vi "Projectile.vi"() -> ()   [LabVIEW 2014]
uses:
  <vilib>/imath/engines/lvmath2/RunTimeEngine/Managers/WorkSpace/UID Generator.vi
  <vilib>/imath/engines/lvmath2/RunTimeEngine/RunTimeType/NIMS_RunTimeType_From StrictType (excl LVString).vi
  <instcachedir>/0/NIMS_RunTimeType_From StrictType (excl LVString)_15A5391EEA9C4AACB9955AC755B83D29.lvgen/NIMS_RunTimeType_From StrictType (excl LVString)_15A5391EEA9C4AACB9955AC755B83D29_000.vi
  <vilib>/imath/engines/lvmath2/RunTimeEngine/LocalVariableDefStatement/MC_LocalVariableDefStatement_Display.vi
  <vilib>/imath/engines/lvmath2/RunTimeEngine/Managers/SymbolTable/Clear UID.vi
  <vilib>/imath/engines/lvmath2/RunTimeEngine/NodeEndStatement/NIMS_NodeEndStatement_Output.vi
  <instcachedir>/0/NIMS_NodeEndStatement_Output_53EC0D466D134D7ABD903AC30B43404B.lvgen/NIMS_NodeEndStatement_Output_53EC0D466D134D7ABD903AC30B43404B_005.vi
  <vilib>/imath/engines/lvmath2/RunTimeEngine/ErrorHandling/NIMS_Finalize Error.vi
  <vilib>/imath/engines/lvmath2/RunTimeEngine/Managers/SymbolTable/NIMS_WorkSpace.lvlib
panel:
  in  "Launch Parameters":T1
  out "Output Cluster":cluster{"Angle (deg)":dbl[], "Range (m)":dbl[]}
  out "XY Graph":cluster{"theta":dbl[], "R":dbl[]}(graph)
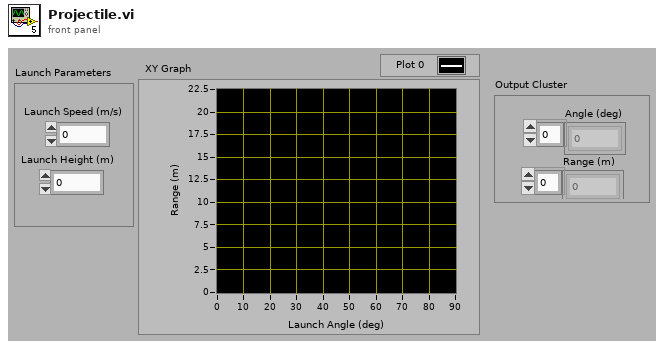
[diagram p1: front panel]
types:
  T1 = cluster{"Launch Speed (m/s)":dbl, "Launch Height (m)":dbl}
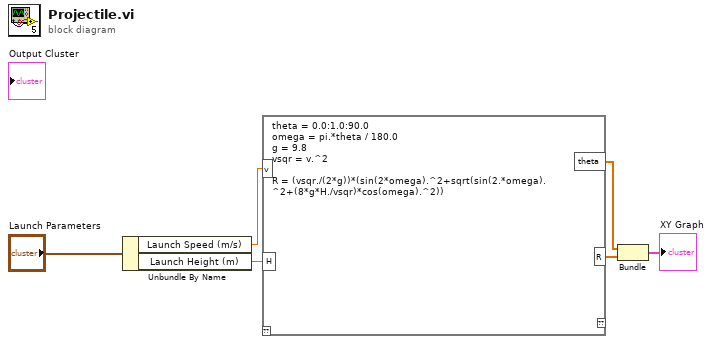
[diagram p0: block diagram]
diagram:
  n1 = Unbundle By Name("Launch Parameters") -> ("Launch Speed (m/s)"=w2:dbl, "Launch Height (m)"=w1:dbl)
  n2 = mathscript code="theta = 0.0:1.0:90.0\nomega = pi.*theta / 180.0\ng = 9.8\nvsqr = v.^2\n\nR = (vsqr./(2*g))*(sin(2*omega).^2+sqrt(sin(2.*omega).^2+(8*g*H./vsqr)*cos(omega).^2))"("v"=w2, "H"=w1) -> ("R"=w6:dbl[], "theta"=w4:dbl[])  [unwired: 1 in, 1 out]
  n3 = Bundle("theta"=w4, "R"=w6) -> (→"XY Graph":cluster{"theta":dbl[], "R":dbl[]})  [unwired: 1 in]
